vi "SeCrTS-DD NS Data.vi"(8 "error in":errorcluster, 9 "AI_V_Data P\nAI_C_Data P\nAO_Data P\nDO_Data P\nACC_Data P\nTC Data P\nDrive_A_C \nDrive_A_D\nAI_C_Data S\nDO_Data S\nAI_V_Rms_P":refnum<queue>[](array[refnum]), 10 "data out":string, 11 "DI P\nDI S":refnum<queue>[](array[refnum])) -> (0 "error out":errorcluster)   [LabVIEW 2022 SP3]
panel:
  out "overflow? 10":bool
  out "overflow? 9":bool
  out "overflow? 8":bool
  out "overflow? 7":bool
  out "overflow? 6":bool
  out "overflow? 5":bool
  out "overflow? 4":bool
  out "overflow? 3":bool
  out "overflow? 2":bool
  out "overflow?":bool
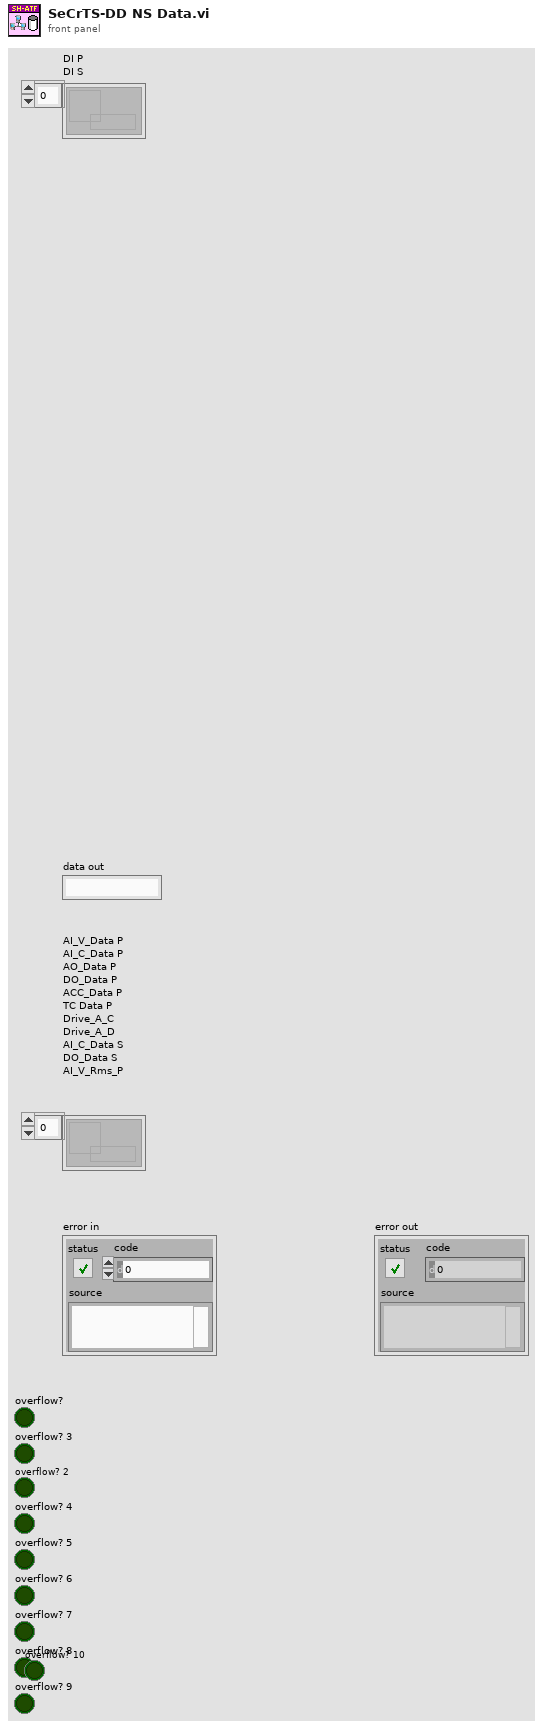
[diagram p1: front panel]
types:
  T1 = cluster{"AI_V_Data":waveform(dbl)[][], "AI_C_Data":waveform(dbl)[][], "AO_Data":waveform(dbl)[][], "DO_Data":waveform(dbl)[][], "DI_Data":digitalwaveform[][], "ACC_Data":waveform(dbl)[][], "TC Data":waveform(dbl)[][], "Drive_A_C":waveform(dbl)[][], "Drive_A_D":waveform(dbl)[][], "AI_V Rms":waveform(dbl)[][]}
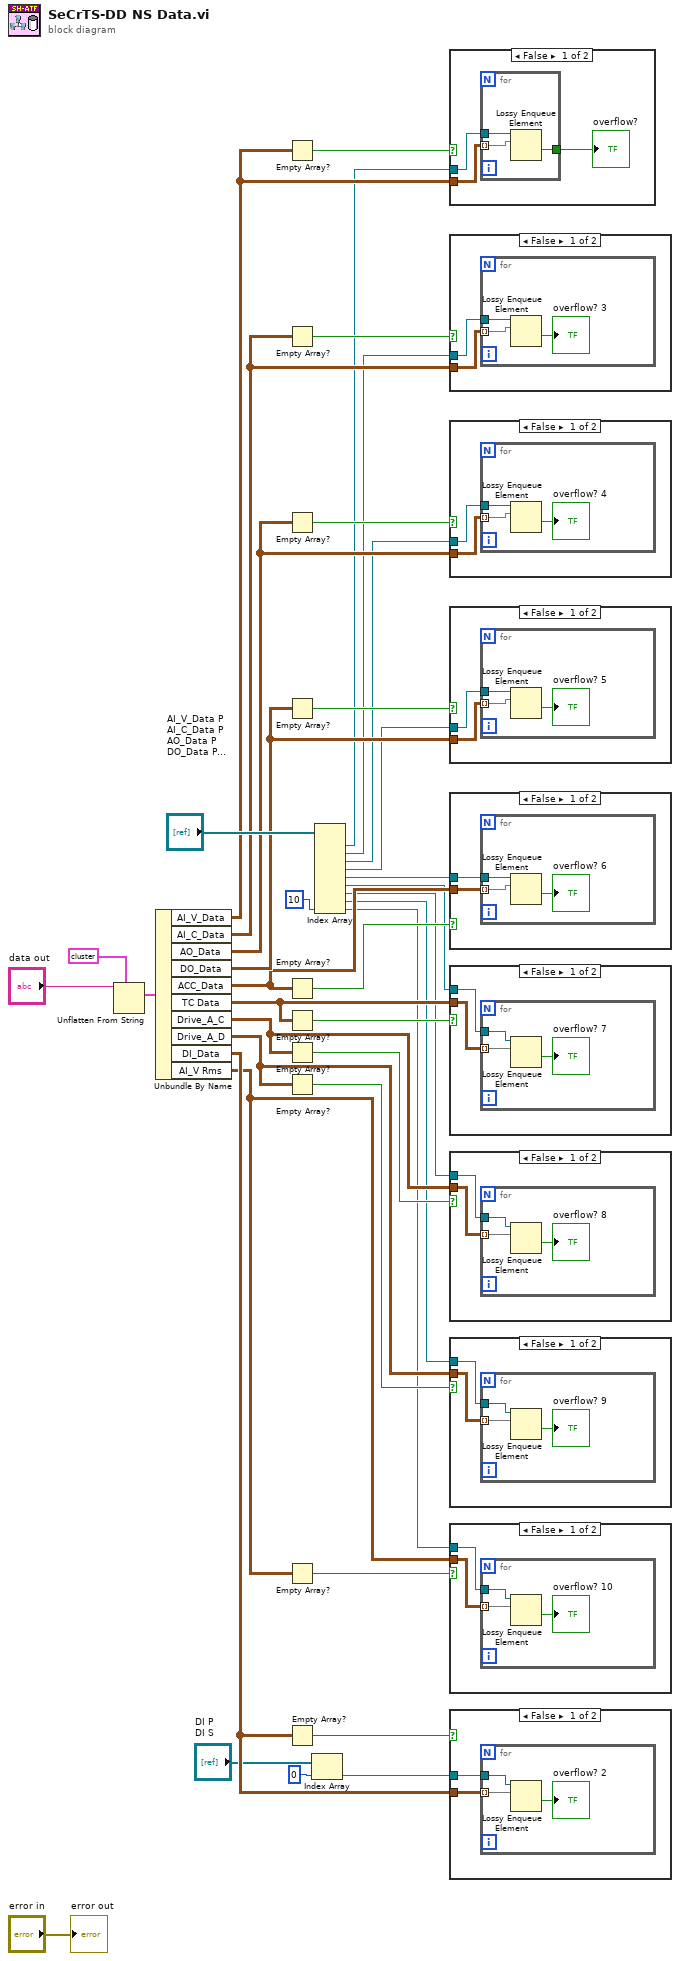
[diagram p0: block diagram]
diagram:
  n1 = Unflatten From String(type=T1 data[101840B] ("data out 2"), binary string="data out") -> (value=w9:T1)  [unwired: 3 in, 2 out]
  n2 = Unbundle By Name(w9) -> ("AI_V_Data"=w32:waveform(dbl)[][], "AI_C_Data"=w34:waveform(dbl)[][], "AO_Data"=w30:waveform(dbl)[][], "DO_Data"=w28:waveform(dbl)[][], "ACC_Data"=w27:waveform(dbl)[][], "TC Data"=w25:waveform(dbl)[][], "Drive_A_C"=w22:waveform(dbl)[][], "Drive_A_D"=w19:waveform(dbl)[][], "DI_Data"=w36:digitalwaveform[][], "AI_V Rms"=w10:waveform(dbl)[][])
  n3 = Empty Array?(array=w32) -> (empty?=w33:bool)
  n4 = Empty Array?(array=w34) -> (empty?=w35:bool)
  n5 = Empty Array?(array=w30) -> (empty?=w31:bool)
  n6 = Empty Array?(array=w28) -> (empty?=w29:bool)
  n7 = Empty Array?(array=w27) -> (empty?=w26:bool)
  n8 = Empty Array?(array=w25) -> (empty?=w24:bool)
  n9 = Empty Array?(array=w22) -> (empty?=w21:bool)
  n10 = Empty Array?(array=w19) -> (empty?=w18:bool)
  n11 = Empty Array?(array=w10) -> (empty?=w11:bool)
  n12 = Empty Array?(array=w36) -> (empty?=w37:bool)
  n13 = Index Array(array="DI P\nDI S", index=0) -> (element=w16:refnum<queue>)
  n14 = Index Array(array="AI_V_Data P\nAI_C_Data P\nAO_Data P\nDO_Data P\nACC_Data P\nTC Data P\nDrive_A_C \nDrive_A_D\nAI_C_Data S\nDO_Data S\nAI_V_Rms_P", index #9=10 ("index")) -> (element #1=w7:refnum<queue>, element #2=w6:refnum<queue>, element #3=w2:refnum<queue>, element #4=w5:refnum<queue>, element #5=w4:refnum<queue>, element #6=w1:refnum<queue>, element #7=w23:refnum<queue>, element #8=w20:refnum<queue>, element #9=w3:refnum<queue>)  [unwired: 8 in]
  n15 = case shown="False" w33 {
    tunnel: w32 -> [w41 _]
    tunnel: w7 -> [w40 _]
    frame False {
      n16 = for {
        tunnel: w41 -> [w42] mode=indexing
        tunnel: w40 -> [w44]
        tunnel: [w43] -> w39
        n17 = Lossy Enqueue Element(queue=w44, element=w42) -> (overflow?=w43:bool)  [unwired: 1 in, 3 out]
      }
      "overflow?" <- w39
    }
    frame True {
    }
  }
  n18 = case shown="False" w35 {
    tunnel: w34 -> [w46 _]
    tunnel: w6 -> [w45 _]
    frame False {
      n19 = for {
        tunnel: w46 -> [w47] mode=indexing
        tunnel: w45 -> [w49]
        n20 = Lossy Enqueue Element(queue=w49, element=w47) -> (overflow?=→"overflow? 3":bool)  [unwired: 1 in, 3 out]
      }
    }
    frame True {
    }
  }
  n21 = case shown="False" w31 {
    tunnel: w30 -> [w51 _]
    tunnel: w2 -> [w50 _]
    frame False {
      n22 = for {
        tunnel: w51 -> [w54] mode=indexing
        tunnel: w50 -> [w53]
        n23 = Lossy Enqueue Element(queue=w53, element=w54) -> (overflow?=→"overflow? 4":bool)  [unwired: 1 in, 3 out]
      }
    }
    frame True {
    }
  }
  n24 = case shown="False" w29 {
    tunnel: w28 -> [w56 _]
    tunnel: w5 -> [w55 _]
    frame False {
      n25 = for {
        tunnel: w56 -> [w57] mode=indexing
        tunnel: w55 -> [w59]
        n26 = Lossy Enqueue Element(queue=w59, element=w57) -> (overflow?=→"overflow? 5":bool)  [unwired: 1 in, 3 out]
      }
    }
    frame True {
    }
  }
  n27 = case shown="False" w26 {
    tunnel: w27 -> [w61 _]
    tunnel: w4 -> [w60 _]
    frame False {
      n28 = for {
        tunnel: w61 -> [w62] mode=indexing
        tunnel: w60 -> [w64]
        n29 = Lossy Enqueue Element(queue=w64, element=w62) -> (overflow?=→"overflow? 6":bool)  [unwired: 1 in, 3 out]
      }
    }
    frame True {
    }
  }
  n30 = case shown="False" w24 {
    tunnel: w25 -> [w66 _]
    tunnel: w1 -> [w65 _]
    frame False {
      n31 = for {
        tunnel: w66 -> [w67] mode=indexing
        tunnel: w65 -> [w69]
        n32 = Lossy Enqueue Element(queue=w69, element=w67) -> (overflow?=→"overflow? 7":bool)  [unwired: 1 in, 3 out]
      }
    }
    frame True {
    }
  }
  n33 = case shown="False" w21 {
    tunnel: w22 -> [w71 _]
    tunnel: w23 -> [w70 _]
    frame False {
      n34 = for {
        tunnel: w71 -> [w72] mode=indexing
        tunnel: w70 -> [w74]
        n35 = Lossy Enqueue Element(queue=w74, element=w72) -> (overflow?=→"overflow? 8":bool)  [unwired: 1 in, 3 out]
      }
    }
    frame True {
    }
  }
  n36 = case shown="False" w18 {
    tunnel: w19 -> [w76 _]
    tunnel: w20 -> [w75 _]
    frame False {
      n37 = for {
        tunnel: w76 -> [w77] mode=indexing
        tunnel: w75 -> [w79]
        n38 = Lossy Enqueue Element(queue=w79, element=w77) -> (overflow?=→"overflow? 9":bool)  [unwired: 1 in, 3 out]
      }
    }
    frame True {
    }
  }
  n39 = case shown="False" w11 {
    tunnel: w10 -> [w81 _]
    tunnel: w3 -> [w80 _]
    frame False {
      n40 = for {
        tunnel: w81 -> [w82] mode=indexing
        tunnel: w80 -> [w84]
        n41 = Lossy Enqueue Element(queue=w84, element=w82) -> (overflow?=→"overflow? 10":bool)  [unwired: 1 in, 3 out]
      }
    }
    frame True {
    }
  }
  n42 = case shown="False" w37 {
    tunnel: w36 -> [w86 _]
    tunnel: w16 -> [w85 _]
    frame False {
      n43 = for {
        tunnel: w86 -> [w87] mode=indexing
        tunnel: w85 -> [w89]
        n44 = Lossy Enqueue Element(queue=w89, element=w87) -> (overflow?=→"overflow? 2":bool)  [unwired: 1 in, 3 out]
      }
    }
    frame True {
    }
  }
  "error out" <- "error in"
